vi "Valid Dip (SubVI).vi"(11 "Lower than Threshold?":bool) -> (0 "Dip Point":u16, 3 "Dip Valid?":bool)   [LabVIEW 2015]
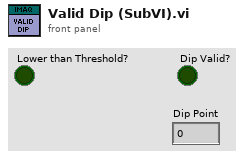
[diagram p1: front panel]
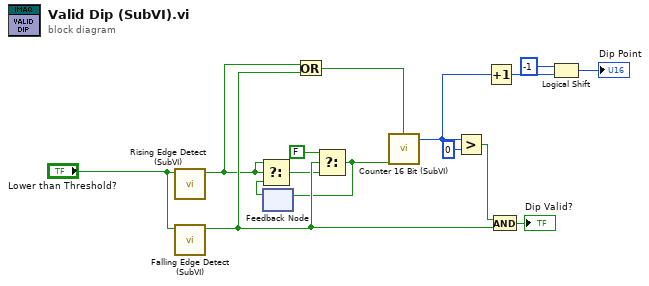
[diagram p0: block diagram]
diagram:
  n1 = call "Rising Edge Detect (SubVI).vi"("Input"="Lower than Threshold?") -> ("Rising Edge?"=w12:bool)  [unwired: 10 in]
  n2 = call "Falling Edge Detect (SubVI).vi"("Input"="Lower than Threshold?") -> ("Falling Edge?"=w13:bool)  [unwired: 10 in]
  n3 = feedback #1() -> (w9:bool)  [unwired: 1 in]
  n4 = Select(t=w12, s=w12, f=w9) -> (s? t:f=w8:bool)
  n5 = Or(x=w12, y=w13) -> (x .or. y?=w14:bool)
  n6 = Select(t=FALSE, s=w13, f=w8) -> (s? t:f=w10:bool)
  n7 = feedback-in #1(w10) -> ()
  n8 = call "Counter 16 Bit (SubVI).vi"("RESET"=w14, "Enable"=w10) -> ("Count"=w4:u16)  [unwired: 11 in, 2 out]
  n9 = Greater?(x=w4, y=u16 0) -> (0:w11:bool)
  n10 = Increment(x=w4) -> (x+1=w1:u16)
  n11 = And(x=w11, y=w13) -> (x .and. y?=→"Dip Valid?":bool)
  n12 = Logical Shift(y=i16 -1, x=w1) -> (x << y=→"Dip Point":u16)
